vi "Create Message Types and Converters.vi"(5 "Enum parameters":T1[](array[typedef]), 7 "Message parameters":T2[](array[typedef]), 8 "error in (no error)":errorcluster, 11 "Library in":refnum<vi>) -> (0 "error out":errorcluster, 3 "Library out":refnum<vi>)   [LabVIEW 2019, in "gRPC Template Creation Utility.lvlib"]
uses:
  gRPC Template Creation Utility.lvlib
  TypeDefs/Message Metadata (Scripting).ctl
  TypeDefs/Message Element Metadata (Scripting).ctl
  TypeDefs/Message Element Type.ctl
  TypeDefs/Enum Metadata (Scripting).ctl
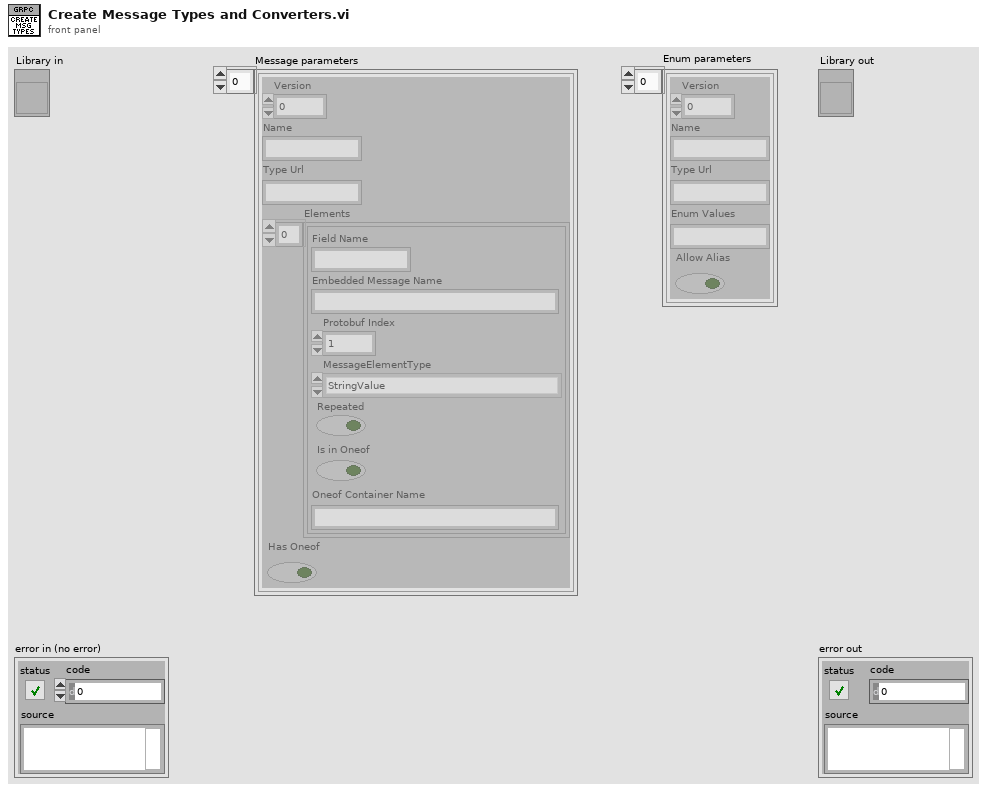
[diagram p1: front panel]
types:
  T1 = typedef "gRPC Template Creation Utility.lvlib/Enum Metadata (Scripting).ctl" = cluster{"Version":i32, "Name":string, "Type Url":string, "Enum Values":string, "Allow Alias":bool}
  T2 = typedef "gRPC Template Creation Utility.lvlib/Message Metadata (Scripting).ctl" = cluster{"Version":i32, "Name":string, "Type Url":string, "Elements":T3[], "Has Oneof":bool}
  T3 = typedef "gRPC Template Creation Utility.lvlib/Message Element Metadata (Scripting).ctl" = cluster{"Field Name":string, "Embedded Message Name":string, "Protobuf Index":i32, "MessageElementType":T4, "Repeated":bool, "Is in Oneof":bool, "Oneof Container Name":string}
  T4 = typedef "gRPC Template Creation Utility.lvlib/Message Element Type.ctl" = enum32{"Int32Value", "FloatValue", "DoubleValue", "BoolValue", "StringValue", "MessageValue", "Int64Value", "UInt32Value", "UInt64Value", "EnumValue", "Bytes", "Fixed64", "Fixed32", "SFixed64", "SFixed32", "SInt64", "SInt32"}
  T5 = enum32{"invalid scope", "public", "private", "protected", "community"}
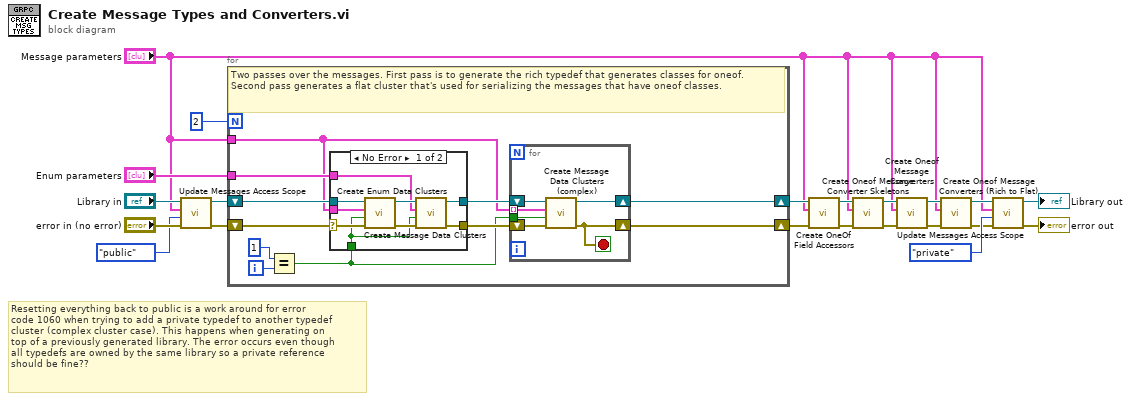
[diagram p0: block diagram]
diagram:
  # "Resetting everything back to public is a work around for error\ncode 1060 when trying to add a private typedef to another typedef\ncluster (complex cluster case). This happens when generating on\ntop of a previously generated library. The error occurs even though \nall typedefs are owned by the same library so a private reference\nshould be fine??"
  n1 = call "Update Messages Access Scope.vi"("error in (no error)"="error in (no error)", "scope"=T5."public", "message parameters"="Message parameters", "library in"="Library in") -> ("error out"=w11:errorcluster, "library out"=w9:refnum<vi>)  [unwired: 6 in]
  n2 = for {
    N: 2 -> [_]
    tunnel: "Enum parameters" -> [w30]
    tunnel: "Message parameters" -> [w24]
    shift-right: [w23] -> w7
    shift-left: w9 -> [w32]
    shift-right: [w22] -> w6
    shift-left: w11 -> [w31]
    i -> [w27]
    # "Two passes over the messages. First pass is to generate the rich typedef that generates classes for oneof. \nSecond pass generates a flat cluster that's used for serializing the messages that have oneof classes."
    n3 = Equal?(x=1, y=w27) -> (x = y?=w25:bool)
    n4 = case shown="No Error" w31 {
      selector: w31 -> [w44 w48]
      tunnel: w24 -> [w41 _]
      tunnel: [w45 w49] -> w29
      tunnel: [w42 w48] -> w28
      tunnel: w32 -> [w47 w49]
      tunnel: w30 -> [w40 _]
      tunnel: w25 -> [w39 _]
      frame No Error {
        n5 = call "Create Message Data Clusters.vi"("error in (no error)"=w44, "Generate_SerializationHelper"=w39, "Message parameters"=w41, "Library"=w47) -> ("error out"=w43:errorcluster, "Library"=w46:refnum<vi>)  [unwired: 6 in]
        n6 = call "Create Enum Data Clusters.vi"("error in (no error)"=w43, "Generate_SerializationHelper"=w39, "Enum parameters"=w40, "Library in"=w46) -> ("error out"=w42:errorcluster, "Library out"=w45:refnum<vi>)  [unwired: 6 in]
      }
      frame Error {
      }
    }
    n7 = for {
      shift-right: [w36] -> w23
      shift-left: w29 -> [w38]
      shift-right: [w34] -> w22
      shift-left: w28 -> [w37]
      tunnel: w24 -> [w35] mode=indexing
      tunnel: w25 -> [w33]
      stop <- w34 stop-if-true
      n8 = call "Create Message Data Clusters (complex).vi"("error in (no error)"=w37, "generate serialization helper"=w33, "message metadata"=w35, "library in"=w38) -> ("error out"=w34:errorcluster, "library out"=w36:refnum<vi>)  [unwired: 6 in]
    }
  }
  n9 = call "Create OneOf Field Accessors.vi"("error in (no error)"=w6, "Message parameters"="Message parameters", "Library in"=w7) -> ("error out"=w14:errorcluster, "Library out"=w15:refnum<vi>)  [unwired: 7 in]
  n10 = call "Create Oneof Message Converter Skeletons.vi"("error in (no error)"=w14, "Message parameters"="Message parameters", "Library in"=w15) -> ("error out"=w19:errorcluster, "Library out"=w18:refnum<vi>)  [unwired: 7 in]
  n11 = call "Create Oneof Message Converters.vi"("error in (no error)"=w19, "Message parameters"="Message parameters", "Library in"=w18) -> ("error out"=w16:errorcluster, "Library out"=w17:refnum<vi>)  [unwired: 7 in]
  n12 = call "Create Oneof Message Converters (Rich to Flat).vi"("error in (no error)"=w16, "Message parameters"="Message parameters", "Library in"=w17) -> ("error out"=w4:errorcluster, "Library out"=w5:refnum<vi>)  [unwired: 7 in]
  n13 = call "Update Messages Access Scope.vi"("error in (no error)"=w4, "scope"=T5."private", "message parameters"="Message parameters", "library in"=w5) -> ("error out"=→"error out":errorcluster, "library out"=→"Library out":refnum<vi>)  [unwired: 6 in]
